vi "Client Forrmat Log.vi"(8 "Params (empty)":string[](array[string]), 9 "Command (\"\")":string, 10 "ServerPort (80)":u16=80, 11 "SERVER (\"\")":string) -> (3 "Log":string[](array[string]))   [LabVIEW 2011]
uses:
  Spartan Client Version.vi
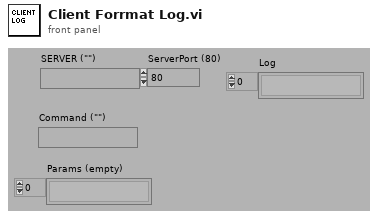
[diagram p1: front panel]
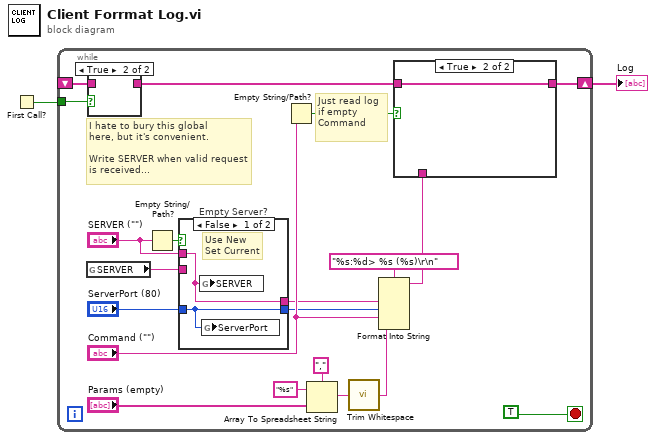
[diagram p0: block diagram]
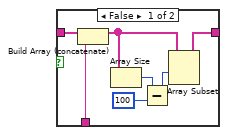
[diagram p3: hidden frame]
diagram:
  n1 = First Call?() -> (First Call?: T/F=w2:bool)
  n2 = while {
    shift-right: [w11] -> w1
    shift-left: _ -> [w13]
    tunnel: w2 -> [w14]
    stop <- TRUE stop-if-true
    # "Just read log\nif empty Command"
    # "I hate to bury this global \nhere, but it's convenient.\n\nWrite SERVER when valid request\nis received..."
    n3 = global read "Spartan Client Version.vi" "SERVER"() -> (w7:string)
    n4 = case shown="True" w14 {
      tunnel: w13 -> [w35 _]
      tunnel: [w35 _] -> w12
      frame False {
      }
      frame True {
      }
    }
    n5 = Empty String/Path?(string/path="SERVER (\"\")") -> (empty?=w8:bool)
    n6 = case "Empty Server?" shown="False" w8 {
      tunnel: w7 -> [_ w26]
      tunnel: "ServerPort (80)" -> [w23 w25]
      tunnel: "SERVER (\"\")" -> [w24 _]
      tunnel: [w24 w26] -> w4
      tunnel: [w23 w25] -> w3
      frame False {
        # "Use New\nSet Current"
        n7 = global write "Spartan Client Version.vi" "SERVER"(w24) -> ()
        n8 = global write "Spartan Client Version.vi" "ServerPort"(w23) -> ()
      }
      frame True {
        # "Use Current"
      }
    }
    n9 = Empty String/Path?(string/path="Command (\"\")") -> (empty?=w10:bool)
    n10 = Array To Spreadsheet String(delimiter (Tab)=",", array="Params (empty)", 3:"%s" ("format string")) -> (spreadsheet string=w18:string)
    n11 = call <vilib>:"Trim Whitespace.vi"("string"=w18) -> ("trimmed string"=w17:string)  [unwired: 1 in]
    n12 = Format Into String(format string="%s:%d> %s (%s)\r\n", w4, w3, "Command (\"\")", w17) -> (resulting string=w21:string)  [unwired: 2 in, 1 out]
    n13 = case shown="True" w10 {
      tunnel: w21 -> [w33 _]
      tunnel: w12 -> [w32 w34]
      tunnel: [w27 w34] -> w11
      frame False {
        n14 = Build Array (concatenate)(w32, w33) -> (w28:string[])
        n15 = Array Size(array=w28) -> (size(s)=w30:i32)
        n16 = Subtract(x=w30, y=100) -> (x-y=w31:i32)
        n17 = Array Subset(array=w28, index=w31) -> (w27:string[])  [unwired: 1 in]
      }
      frame True {
      }
    }
  }
  "Log" <- w1
